vi "TEST - Set Data Name - Attributes.vi"(8 "error in (no error)":errorcluster) -> (0 "error out":errorcluster, 2 "pass":bool)   [LabVIEW 2020, in "test_openg_variant.lvlib"]
uses:
  test_openg_variant.lvlib
  <userlib>/_OpenG.lib/error/error.llb/openg_error.lvlib
  source/library/openg_variant.lvlib
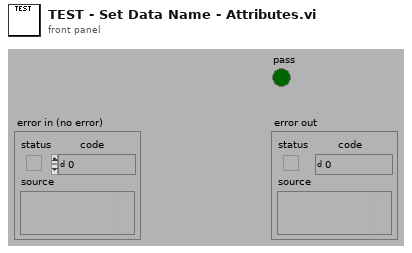
[diagram p1: front panel]
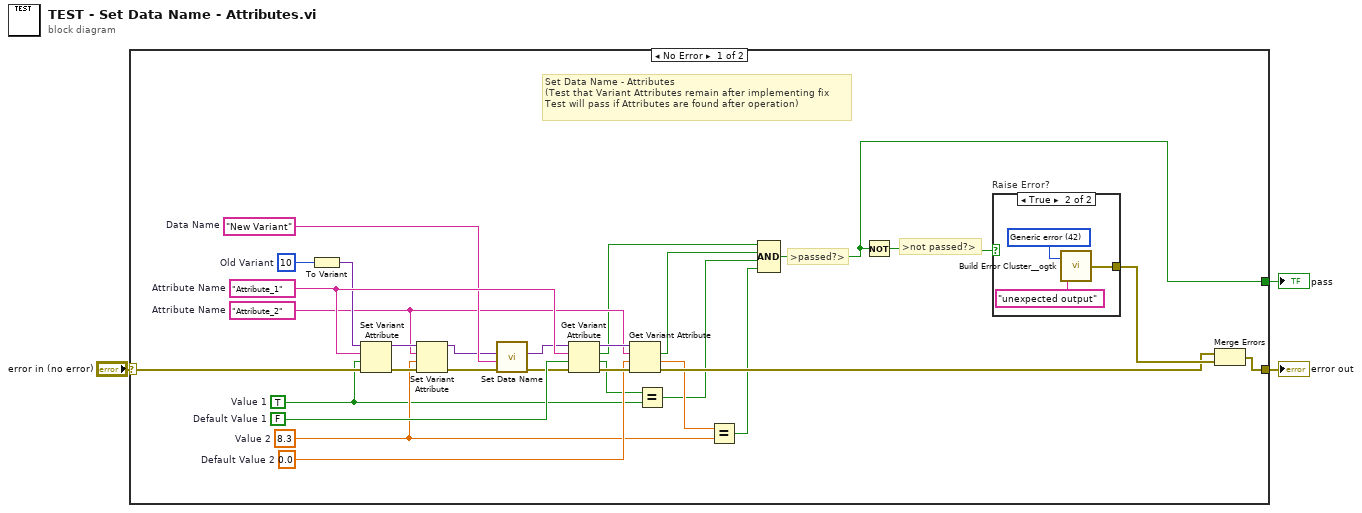
[diagram p0: block diagram]
diagram:
  n1 = case shown="No Error" "error in (no error)" {
    selector: "error in (no error)" -> [w23 w36]
    tunnel: [w10 _] -> w3
    tunnel: [w32 w36] -> w1
    frame No Error {
      w13 = 0.0  # Default Value 2
      w9 = 8.3  # Value 2
      w14 = "Attribute_2"  # Attribute Name
      w27 = 10  # Old Variant
      w29 = FALSE  # Default Value 1
      w6 = TRUE  # Value 1
      w26 = "New Variant"  # Data Name
      w28 = "Attribute_1"  # Attribute Name
      # "Set Data Name - Attributes\n(Test that Variant Attributes remain after implementing fix\nTest will pass if Attributes are found after operation)"
      # ">not passed?>"
      # ">passed?>"
      n2 = To Variant(anything=w27) -> (Variant=w18:variant)
      n3 = Set Variant Attribute(Variant=w18, name=w28, value=w6, error in=w23) -> (Variant out=w19:variant, error out=w22:errorcluster)  [unwired: 1 out]
      n4 = Set Variant Attribute(Variant=w19, name=w14, value=w9, error in=w22) -> (Variant out=w21:variant, error out=w20:errorcluster)  [unwired: 1 out]
      n5 = call "Set Data Name.vi"("error in (no error)"=w20, "Data Name"=w26, "Data"=w21) -> ("error out"=w24:errorcluster, "Renamed Data"=w25:variant)  [unwired: 7 in]
      n6 = Get Variant Attribute(Variant=w25, name=w28, default value (empty Variant)=w29, error in=w24) -> (duplicate Variant=w15:variant, found=w11:bool, value=w7:bool, error out=w17:errorcluster)
      n7 = Get Variant Attribute(Variant=w15, name=w14, default value (empty Variant)=w13, error in=w17) -> (found=w12:bool, value=w8:dbl, error out=w16:errorcluster)  [unwired: 1 out]
      n8 = Equal?(x=w7, y=w6) -> (x = y?=w5:bool)
      n9 = Equal?(x=w8, y=w9) -> (x = y?=w4:bool)
      n10 = Compound Arithmetic op=AND(w11, w12, w5, w4) -> (w10:bool)
      n11 = Not(x=w10) -> (.not. x?=w30:bool)
      n12 = case "Raise Error?" shown="True" w30 {
        tunnel: [_ w33] -> w31
        frame False {
        }
        frame True {
          w34 = 42 items=["No error", "Argument error", "Memory is full", "Out of zone", "End of file", "File already open", "Generic file I/O error", "File not found", "File permission error", "Disk is full", "Duplicate path", "Too many files open", "System feature not enabled", "Resource file not found", "Cannot add resource", "Resource not found", "Image not found", "Image memory error", "Pen does not exist", "Config type invalid", "Config token not found", "Config parse error", "Config memory error", "Bad external code format", "Bad external code offset", "External code not present", "Null window", "Destroy window error", "Null menu", "Print aborted", "Bad print record", "Print driver error", "Windows error during printing", "Memory error during printing", "Print dialog error", "Generic print error", "Invalid device refnum", "Device not found", "Device parameter error", "Device unit error", "Cannot open device", "Device call aborted", "Generic error", "Cancelled by user", "Object ID too low", "Object ID too high", "Object not in heap", "Unknown heap", "Unknown object (invalid DefProc)", "Unknown object (DefProc not in table)", "Message out of range", "Invalid (null) method", "Unknown message", "Manager call not supported", "Bad address", "Network operation in progress", "Network operation timed out", "Connection is busy", "Network attribute not supported", "Network error", "Address in use", "System out of memory", "Connection aborted", "Connection refused", "Not connected", "Already connected", "Connection closed", "Initialization error (interapplication manager)", "Bad occurrence", "Wait on unbound occurrence handler", "Occurrence queue overflow", "Datalog type conflict", "Unused", "Unrecognized type (interapplication manager)", "Memory corrupt", "Failed to make temporary DLL", "Old CIN version", "Drag socket not found", "Failed to load drop-object", "Failed to register OLE object", "Failed to release OLE object", "Format specifier type mismatch", "Unknown format specifier", "Too few format specifiers", "Too many format specifiers", "Scan failed", "Newer CIN version", "Error converting to variant", "Runtime menu error", "Password tampered", "Variant attribute not found", "Incompatible variant data type", "Event data is not available", "Event Store is not present", "Occurrence is not found", "Event Queue is not created", "Event info is not available", "Refnum passed is NULL", "Error retrieving Class GUID", "Error retrieving CoClass GUID", "Error retrieving TypeLib GUID.", "Bad built application magic bytes.", "Specific driver is different from the specific driver associated with the Logical Name.", "There is no session opened to the class driver.", "Max Error", "MAX - Error with config objects", "MAX - Error loading configuration", "MAX - Group not supported"]
          n13 = call <userlib>:"Build Error Cluster__ogtk.vi"("String to Prepend to source (\"\")"="unexpected output" ("String to Prepend to source (\"\")"), "code"=w34) -> ("error out"=w33:errorcluster)
        }
      }
      n14 = Merge Errors(w16, w31) -> (w32:errorcluster)
    }
    frame Error {
    }
  }
  "pass" <- w3
  "error out" <- w1
